vi "database_connection_write_dev_MQTT_database_array.vi"(8 "error in (no error)":errorcluster, 9 "data 2":dbl[](array[numeric]), 10 "Machine Data":T5={"Zload"="", "Yload"="", "Xload"="", "path_position"="", "Fovr"="", "SspeedOvr"="", "Program Name"="", "Program status"="", "Block of code being executed"="", "Line of code"="", "Machine availability"="", "Emergency status"="", "Controller mode"="", "Tool_id"="UNAVAILABLE"}, 11 "current time 2":timestamp) -> (3 "error out":errorcluster)   [LabVIEW 2017]
uses:
  mqtt Folder/src/class/mqtt/mqttTypedef/mqttConnectionStatus.ctl
  mqtt Folder/src/class/mqtt/mqttTypedef/mqttConnectionMeta.ctl
  mqtt Folder/src/class/mqtt/mqttTypedef/mqttQOSlevel.ctl
  data_base_structure.ctl
  mqtt Folder/src/class/mqtt/mqttConfigFunction.ctl
  mqtt Folder/src/class/mqtt/mqttTypedef/mqttBroker.ctl
  mqtt Folder/src/class/mqtt/mqttTypedef/mqttConnectionFlags.ctl
  mqtt Folder/src/class/mqtt/mqttTypedef/mqttWillInformation.ctl
  mqtt Folder/src/class/mqtt/mqttTXqueue/mqttTXdataQueueFunction.ctl
  mqtt Folder/src/class/mqtt/mqttTXqueue/mqttRXsubscriptionEventFunction.ctl
  <vilib>/addons/database/Connection.llb/DB Tools Open Connec (Path).vi
  mqtt Folder/src/class/mqtt/mqtt.lvclass
  <vilib>/addons/database/NI_Database_API.lvlib
panel:
  out "output array 2":dbl[](array[numeric])
  out "output cluster 2":T1
  out "output cluster":cluster{"current time 2":timestamp, dbl}
  out "output array":string[](array[string])
  out "size(s) 2":i32
  out "error out 3":errorcluster
  out "publishSuccess 2":bool=TRUE
  out "publishMessageID 2":u16 format="%02x"
  out "valueSent 2":string="14:19:17.238_"
  in  "connMeta 2":T2
  in  "topic 2":string="a/b"
  out "connStatus 2":T4
  out "sessionPresent 2":bool
  out "data 3":dbl[](array[numeric])
  out "size(s)":i32
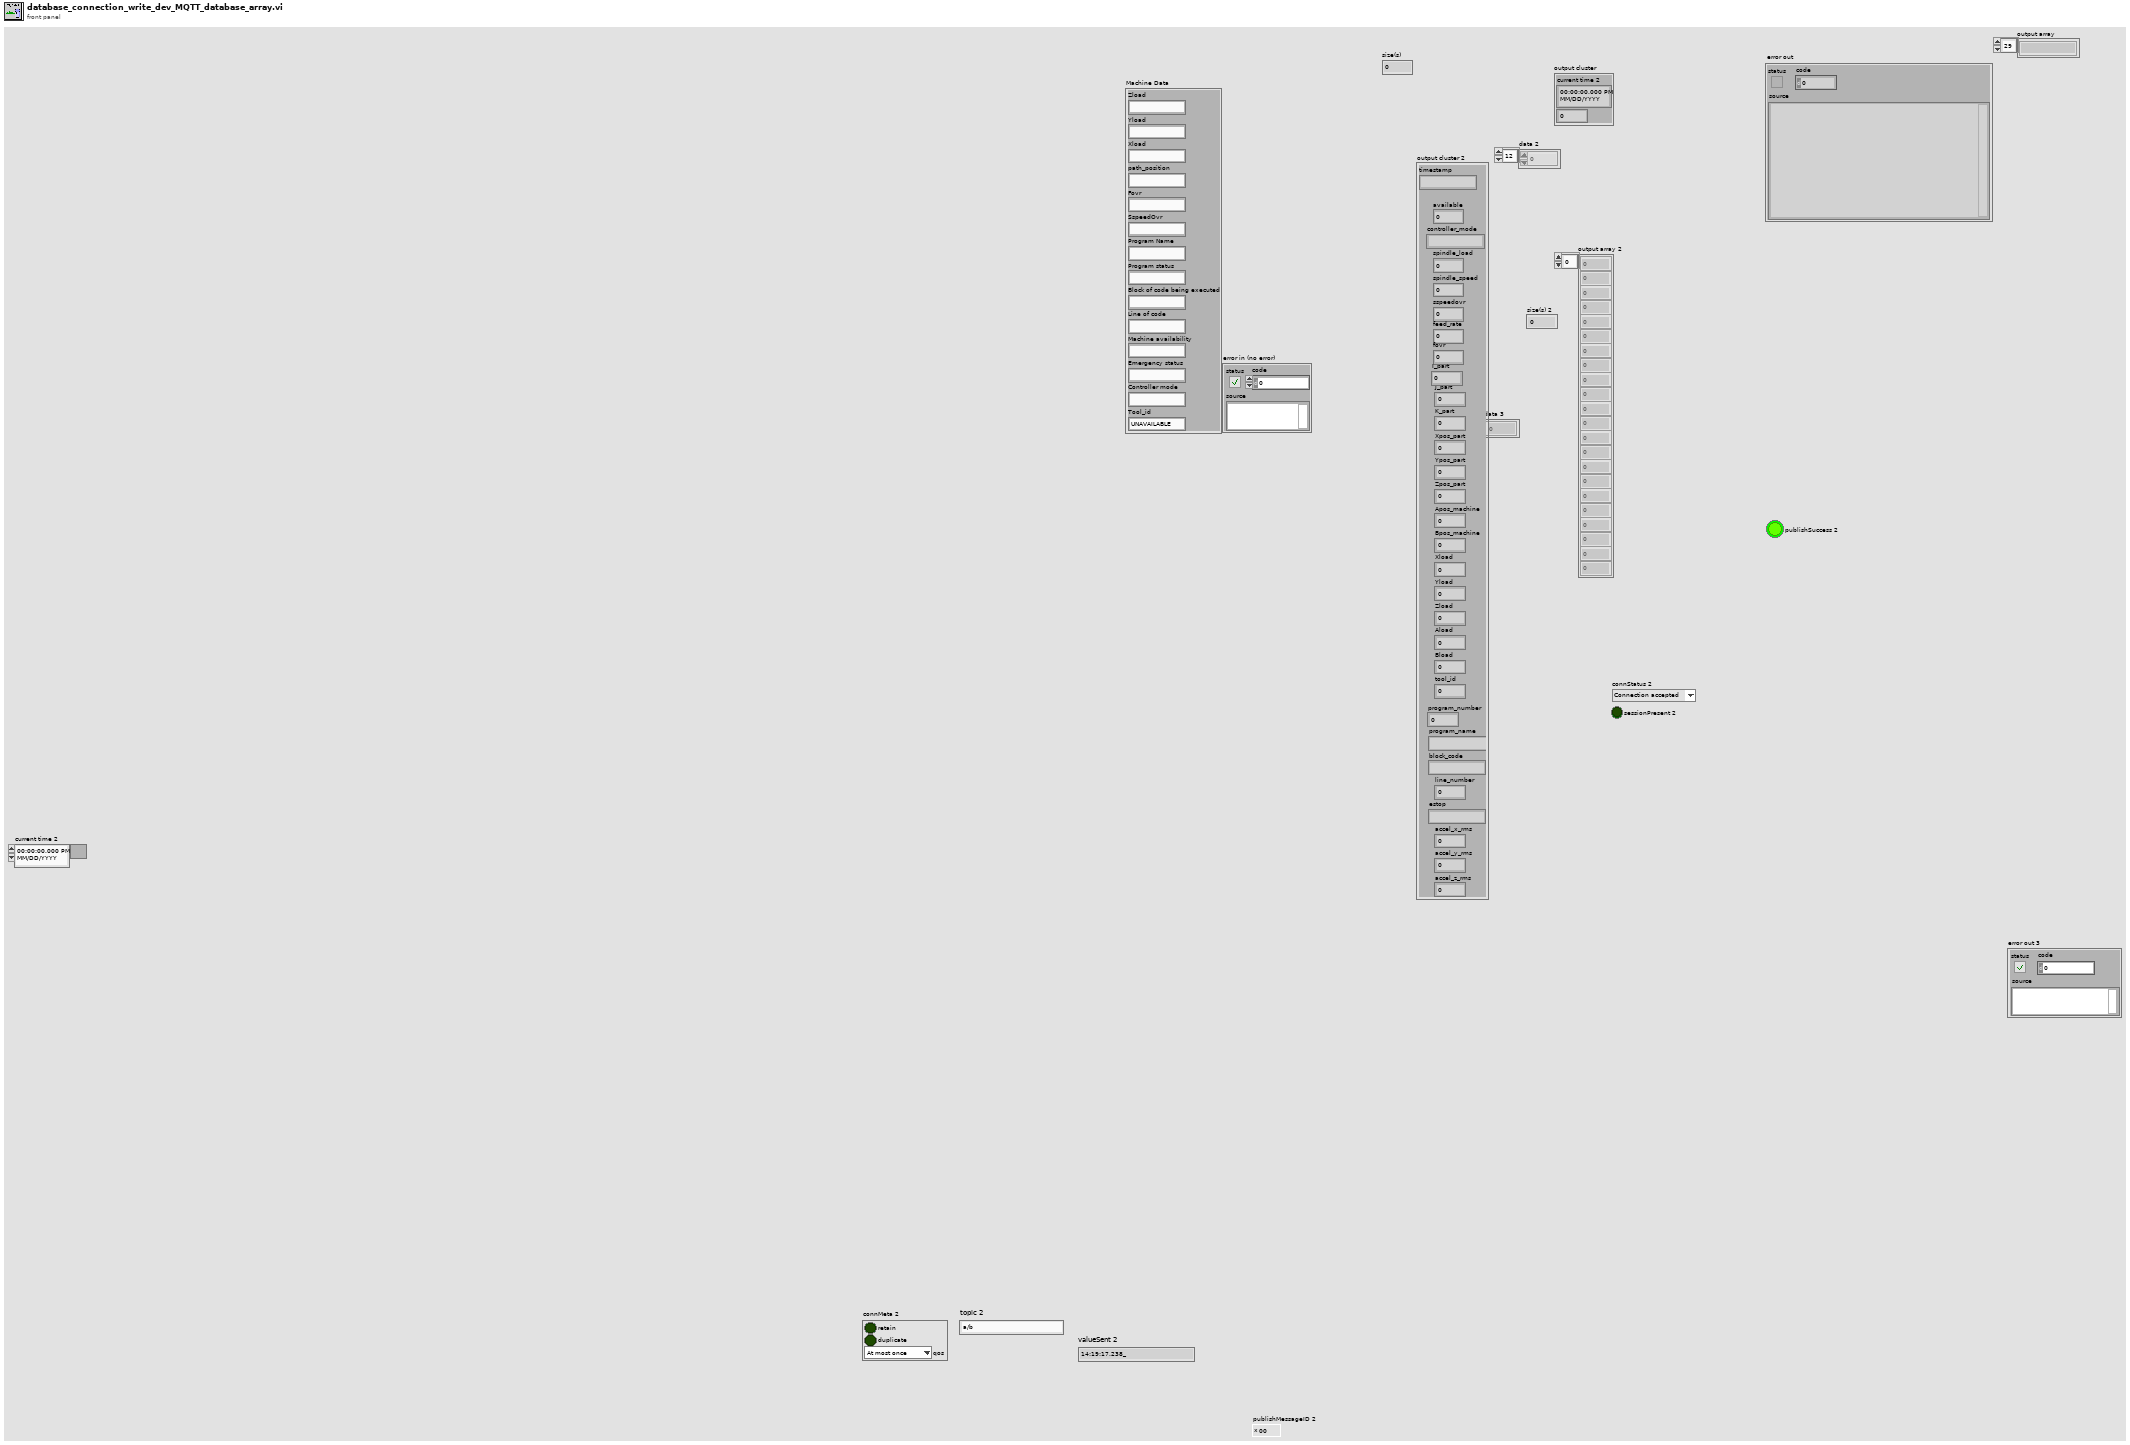
[diagram p1: front panel]
types:
  T1 = typedef "data_base_structure.ctl" = cluster{"available ":dbl, "controller_mode":string, "spindle_load":dbl, "spindle_speed ":dbl, "sspeedovr":dbl, "J_part":dbl, "K_part":dbl, "Xpos_part":dbl, "Ypos_part":dbl, "Zpos_part":dbl, "Apos_machine":dbl, "Bpos_machine":dbl, "Xload":dbl, "Yload":dbl, "Zload":dbl, "Aload":dbl, "Bload":dbl, "tool_id":dbl, "program_name":string, "block_code":string, "line_number":dbl, "estop":string, "accel_x_rms":dbl, "accel_y_rms":dbl, "accel_z_rms":dbl, "program_number":dbl, "timestamp":string, "feed_rate ":dbl, "fovr":dbl, "I_part ":dbl}
  T2 = typedef "mqttConnectionMeta.ctl" = cluster{"retain":bool, "duplicate":bool, "qos":T3}
  T3 = typedef "mqttQOSlevel.ctl" = enum8{"At most once", "At least once", "Exactly once", "Reserved"}
  T4 = typedef "mqttConnectionStatus.ctl" = enum16{"Connection accepted", "Connection refused: unacceptable protocol version", "Connection refused: identifier rejected", "Connection refused: Server unavailable", "Connection refused: bad user name or password", "Connection refused: not authorized"}
  T5 = cluster{"Zload":string, "Yload":string, "Xload":string, "path_position":string, "Fovr":string, "SspeedOvr":string, "Program Name":string, "Program status":string, "Block of code being executed":string, "Line of code":string, "Machine availability":string, "Emergency status":string, "Controller mode":string, "Tool_id":string}
  T6 = typedef "mqttRXsubscriptionEventFunction.ctl" = enum16{"init", "deinit", "getEventRef", "event"}
  T7 = typedef "mqttTXdataQueueFunction.ctl" = enum16{"init", "deinit", "getQueue", "enqueue"}
  T8 = typedef "mqttWillInformation.ctl" = cluster{"User Name":string, "Password":string}
  T9 = typedef "mqttConnectionFlags.ctl" = cluster{"reserved":bool, "clean session":bool, "will flag":bool, "willQOS":enum8{"At most once", "At least once", "Exactly once", "Reserved"}, "will retain":bool, "password":bool, "user name":bool}
  T10 = typedef "mqttBroker.ctl" = cluster{"address":string, "port":u16, "connTimeout":i32, "writeTimeout":i32, "readTimeout":i32, "subTimeout":i32}
  T11 = typedef "mqtt.lvclass/mqttConfigFunction.ctl" = enum16{"init", "deinit", "set", "get"}
  T12 = enum8{"Enabled", "Disabled", "Disabled and Grayed Out"}
  T13 = cluster{"data 2[0]":dbl, "data 2[1]":dbl, "data 2[2]":dbl, "data 2[3]":dbl, "data 2[4]":dbl, "data 2[5]":dbl, "data 2[6]":dbl, "data 2[7]":dbl, "data 2[8]":dbl, "data 2[9]":dbl, "data 2[10]":dbl, "data 2[11]":dbl, "data 2[12]":dbl, "data 2[13]":dbl, "data 2[14]":dbl, "data 2[15]":dbl, "data 2[16]":dbl, "data 2[17]":dbl}
  T14 = cluster{"data 2[0]":dbl, "data 2[1]":dbl, "data 2[2]":dbl, "data 2[3]":dbl, "data 2[4]":dbl, "data 2[5]":dbl, "data 2[6]":dbl, "data 2[7]":dbl, "data 2[8]":dbl, "data 2[9]":dbl, "data 2[10]":dbl, "data 2[11]":dbl, "data 2[12]":dbl, "data 2[13]":dbl, "data 2[14]":dbl, "data 2[15]":dbl, "data 2[16]":dbl, "data 2[17]":dbl, "data 2[18]":dbl, "data 2[19]":dbl, "data 2[20]":dbl, "data 2[21]":dbl}
  T15 = typedef "NI_Database_API.lvlib/Conn ObjectReference.ctl" = refnum<k1>
  T16 = cluster{"date/time string":string, dbl, "Controller mode":string, "data 2[0]":dbl, "data 2[1]":dbl, "data 2[2]":dbl, "data 2[3]":dbl, "data 2[4]":dbl, "data 2[5]":dbl, "data 2[6]":dbl, "data 2[7]":dbl, "data 2[8]":dbl, "data 2[9]":dbl, "data 2[10]":dbl, "data 2[11]":dbl, "data 2[12]":dbl, "data 2[13]":dbl, "data 2[14]":dbl, "data 2[15]":dbl, "data 2[16]":dbl, "data 2[17]":dbl, dbl, "data 2[18]":dbl, "Program Name":string, "Block of code being executed":string, dbl, "Emergency status":string, "data 2[20]":dbl, "data 2[19]":dbl, "data 2[21]":dbl}
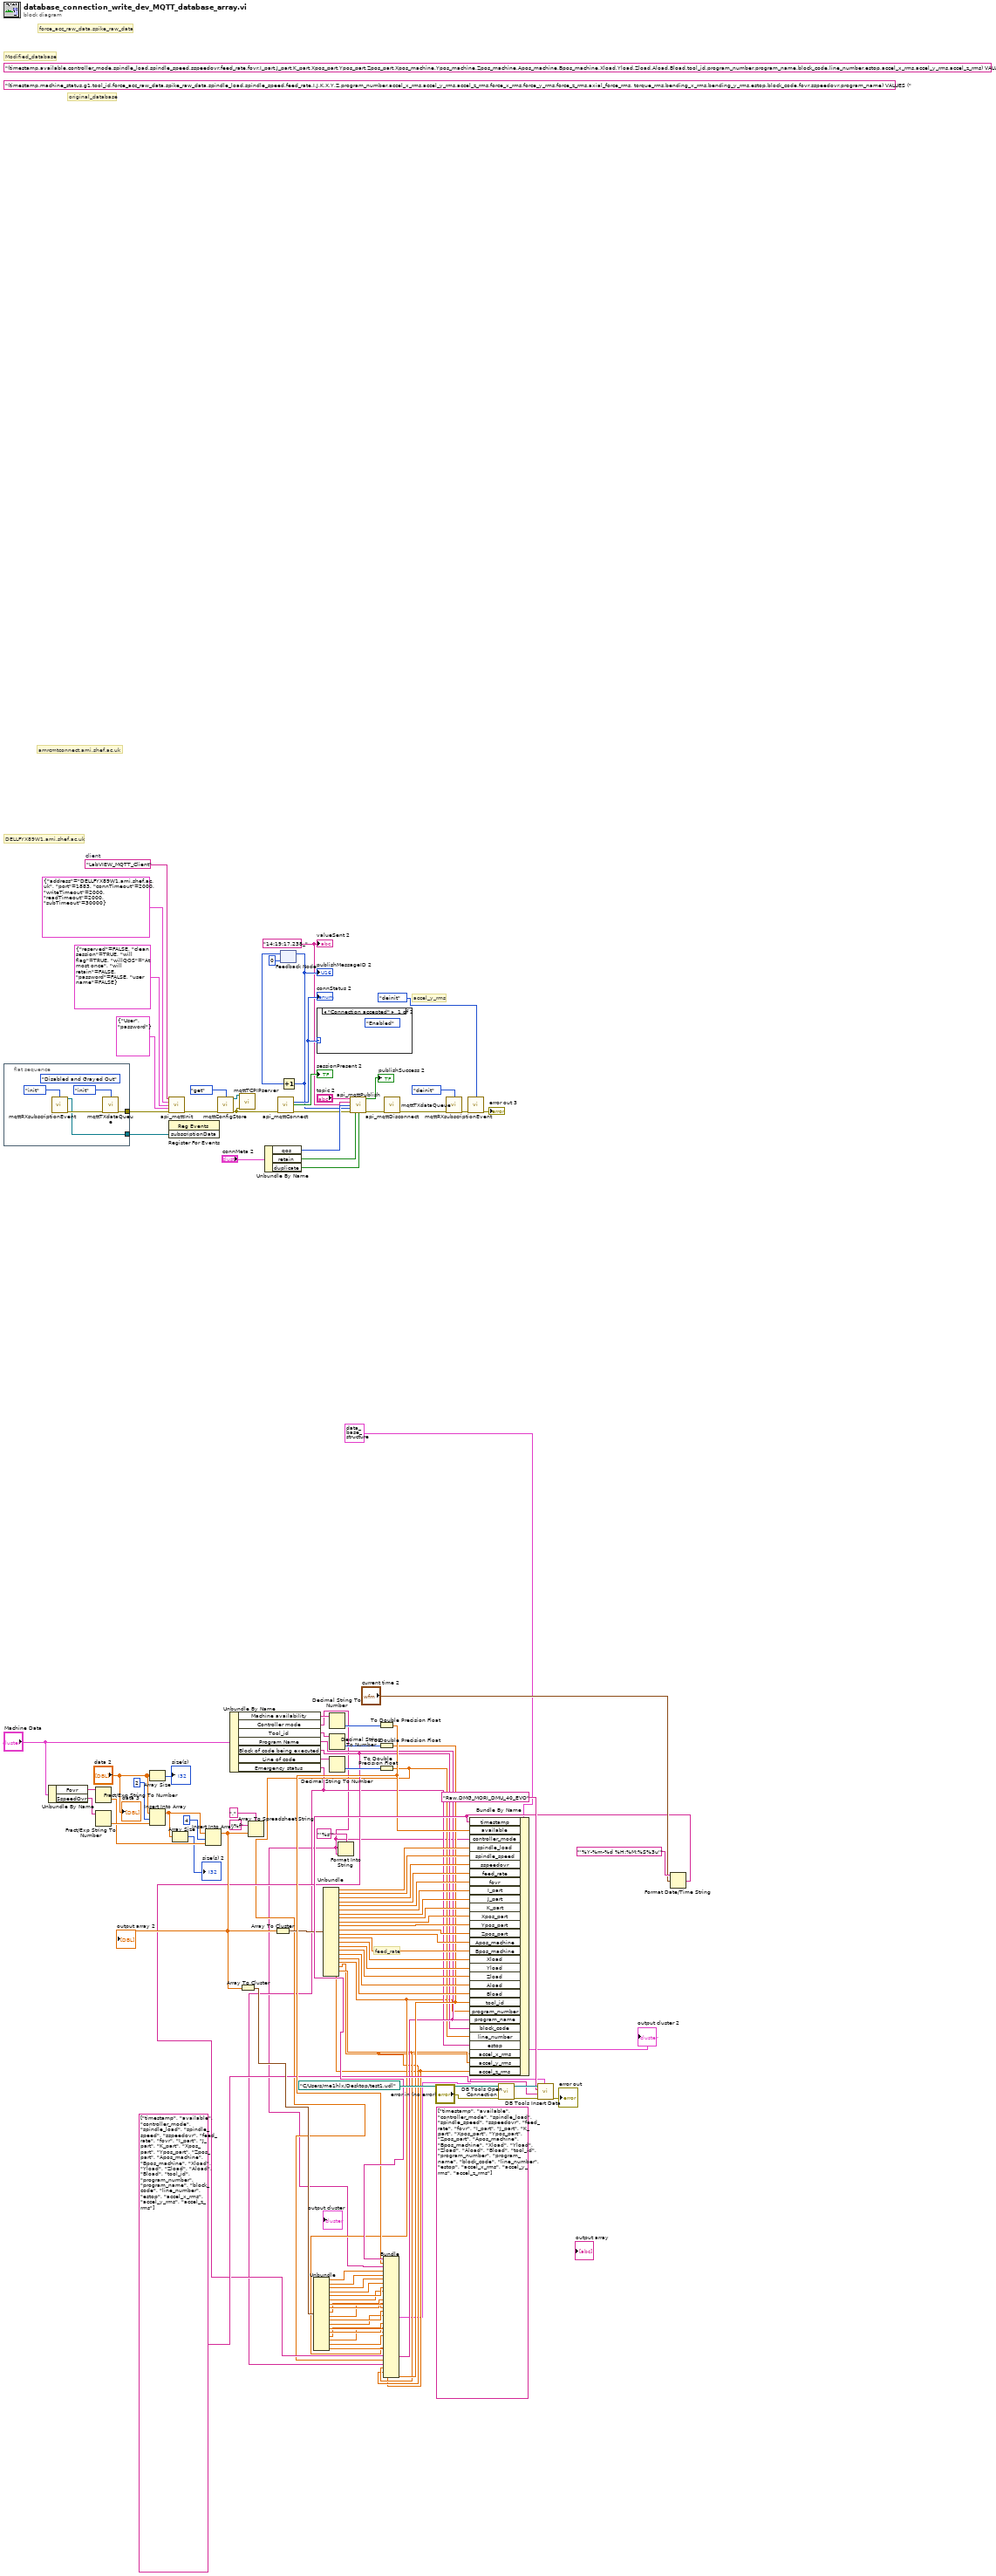
[diagram p0: block diagram]
diagram:
  (unwired) string[] ["timestamp", "available", "controller_mode", "spindle_load", "spindle_speed", "sspeedovr", "feed_rate", "fovr", "I_part", "J_part", "K_part", "Xpos_part", "Ypos_part", "Zpos_part", "Apos_machine", "Bpos_machine", "Xload", "Yload", "Zload", "Aload", "Bload", "tool_id", "program_number", "program_name", "block_code", "line_number", "estop", "accel_x_rms", "accel_y_rms", "accel_z_rms"]
  w71 = "14:19:17.238_" ("valueSent 2")
  (unwired) "(timestamp,available,controller_mode,spindle_load,spindle_speed,sspeedovr,feed_rate,fovr,I_part,J_part,K_part,Xpos_part,Ypos_part,Zpos_part,Xpos_machine,Ypos_machine,Zpos_machine,Apos_machine,Bpos_machine,Xload,Yload,Zload,Aload,Bload,tool_id,program_number,program_name,block_code,line_number,estop,accel_x_rms,accel_y_rms,accel_z_rms) VALUES (" ("string")
  w104 = "LabVIEW_MQTT_Client"  # client
  (unwired) "(timestamp,machine_status,g1,tool_id,force_acc_raw_data,spike_raw_data,spindle_load,spindle_speed,feed_rate,I,J,K,X,Y,Z,program_number,accel_x_rms,accel_y_rms,accel_z_rms,force_x_rms,force_y_rms,force_z_rms,axial_force_rms, torque_rms,bending_x_rms,bending_y_rms,estop,block_code,fovr,sspeedovr,program_name) VALUES (" ("string")
  # "accel_y_rms"
  # "feed_rate"
  # "original_database"
  # "force_acc_raw_data,spike_raw_data"
  # "Modified_database"
  # "amrcmtconnect.ami.shef.ac.uk"
  # "DELLFYX89W1.ami.shef.ac.uk"
  n1 = flat-sequence {
    tunnel: [w116] -> w109
    tunnel: [w113] -> w105
    frame #0 {
      (unwired) T12."Disabled and Grayed Out" ("Disabled")
      n2 = call "mqttRXsubscriptionEvent.vi"("function"=mqttRXsubscriptionEventFunction."init") -> ("subscriptionData"=w113:refnum<user-event>, "error out"=w115:errorcluster)  [unwired: 13 in]
      n3 = call "mqttTXdataQueue.vi"("function"=mqttTXdataQueueFunction."init", "error in (no error)"=w115) -> ("error out"=w116:errorcluster)  [unwired: 12 in, 1 out]
    }
  }
  n4 = Unbundle By Name("Machine Data") -> ("Fovr"=w75:string, "SspeedOvr"=w80:string)
  n5 = Fract/Exp String To Number(string=w75) -> (number=w77:dbl)  [unwired: 3 in, 1 out]
  n6 = Fract/Exp String To Number(string=w80) -> (number=w79:dbl)  [unwired: 3 in, 1 out]
  n7 = Array Size(array="data 2") -> (size(s)=→"size(s)":i32)
  n8 = Insert Into Array(array="data 2", index=2, new element=w79) -> (w67:dbl[])
  n9 = call "api_mqttInit.vi"("client"=w104, "broker"=T10 {"address"="DELLFYX89W1.ami.shef.ac.uk", "port"=1883, "connTimeout"=2000, "writeTimeout"=2000, "readTimeout"=2000, "subTimeout"=30000}, "connFlags"=T9 {"reserved"=FALSE, "clean session"=TRUE, "will flag"=TRUE, "willQOS"=enum."At most once", "will retain"=FALSE, "password"=FALSE, "user name"=FALSE}, "User Info"=T8 {"User Name"="User", "Password"="password"}, "error in (no error)"=w109) -> ("error out"=w107:errorcluster)  [unwired: 10 in]
  n10 = register-events(w105) -> ()  [unwired: 2 in, 2 out]
  n11 = Array Size(array=w67) -> (size(s)=→"size(s) 2":i32)
  n12 = Insert Into Array(array=w67, index=4, new element=w77) -> (w30:dbl[])
  "output array 2" <- w30
  n13 = call "mqttConfigStore.vi"("function"=mqttConfigFunction."get", "error in (no error)"=w107) -> ("mqtt.lvclass out"=w106:refnum<class "mqtt.lvclass">, "error out"=w98:errorcluster)  [unwired: 12 in]
  n14 = Unbundle By Name("Machine Data") -> ("Machine availability"=w40:string, "Controller mode"=w3:string, "Tool_id"=w62:string, "Program Name"=w11:string, "Block of code being executed"=w10:string, "Line of code"=w61:string, "Emergency status"=w8:string)
  n15 = call "mqttTCPIPserver.vi"("mqtt.lvclass"=w106, "error in (no error)"=w98) -> ()  [unwired: 12 in, 2 out]
  n16 = Array To Cluster(array=w30) -> (cluster=w29:T13)
  n17 = Array To Spreadsheet String(delimiter (Tab)=",", array=w30, 3:"%f" ("format string")) -> ()  [unwired: 1 out]
  n18 = Unbundle By Name("connMeta 2") -> ("qos"=w95:T3, "retain"=w94:bool, "duplicate"=w93:bool)
  n19 = Array To Cluster(array=w30) -> (cluster=w34:T14)
  n20 = call "api_mqttConnect.vi"("error in (no error)"=w98) -> ("connStatus"=w100:T4, "sessionPresent"=→"sessionPresent 2":bool, "error out"=w92:errorcluster)  [unwired: 11 in, 1 out]
  "connStatus 2" <- w100
  n21 = feedback #1(u16 0) -> (w90:u16)
  n22 = Increment(x=w90) -> (x+1=w89:u16)
  "publishMessageID 2" <- w89
  n23 = feedback-in #1(w89) -> ()
  n24 = Unbundle(w29) -> ("data 2[0]"=w33:dbl, "data 2[1]"=w32:dbl, "data 2[2]"=w31:dbl, "data 2[3]"=w28:dbl, "data 2[4]"=w26:dbl, "data 2[5]"=w25:dbl, "data 2[6]"=w24:dbl, "data 2[7]"=w23:dbl, "data 2[8]"=w22:dbl, "data 2[9]"=w21:dbl, "data 2[10]"=w20:dbl, "data 2[11]"=w19:dbl, "data 2[12]"=w18:dbl, "data 2[13]"=w17:dbl, "data 2[14]"=w16:dbl, "data 2[15]"=w15:dbl, "data 2[16]"=w14:dbl, "data 2[17]"=w13:dbl)
  n25 = case shown="\"Connection accepted\"" w100 {
    frame "Connection accepted" {
      (unwired) T12."Enabled" ("Disabled")
    }
    frame Default {
    }
  }
  n26 = Unbundle(w34) -> ("data 2[0]"=w57:dbl, "data 2[1]"=w56:dbl, "data 2[2]"=w55:dbl, "data 2[3]"=w54:dbl, "data 2[4]"=w53:dbl, "data 2[5]"=w52:dbl, "data 2[6]"=w51:dbl, "data 2[7]"=w50:dbl, "data 2[8]"=w49:dbl, "data 2[9]"=w48:dbl, "data 2[10]"=w47:dbl, "data 2[11]"=w46:dbl, "data 2[12]"=w45:dbl, "data 2[13]"=w44:dbl, "data 2[14]"=w66:dbl, "data 2[15]"=w43:dbl, "data 2[16]"=w65:dbl, "data 2[17]"=w42:dbl, "data 2[18]"=w7:dbl, "data 2[19]"=w5:dbl, "data 2[20]"=w6:dbl, "data 2[21]"=w4:dbl)
  n27 = Decimal String To Number(string=w40) -> (number=w39:i32)  [unwired: 2 in, 1 out]
  n28 = Decimal String To Number(string=w62) -> (number=w63:i32)  [unwired: 2 in, 1 out]
  n29 = Decimal String To Number(string=w61) -> (number=w60:i32)  [unwired: 2 in, 1 out]
  n30 = Format Into String(format string="'%s'", w3) -> ()  [unwired: 2 in, 2 out]
  n31 = call "api_mqttPublish.vi"("topic"="topic 2", "value"=w71, "QoS (At most once)"=w95, "messageID"=w89, "error in (no error)"=w92, "retain(F)"=w94, "duplicate(F)"=w93) -> ("success"=→"publishSuccess 2":bool, "error out"=w82:errorcluster)  [unwired: 7 in]
  n32 = To Double Precision Float(number=w39) -> (double precision float=w36:dbl)
  n33 = To Double Precision Float(number=w63) -> (double precision float=w12:dbl)
  n34 = To Double Precision Float(number=w60) -> (double precision float=w9:dbl)
  n35 = call "api_mqttDisconnect.vi"("error in (no error)"=w82) -> ("error out"=w86:errorcluster)  [unwired: 13 in, 1 out]
  n36 = call "mqttTXdataQueue.vi"("function"=mqttTXdataQueueFunction."deinit", "error in (no error)"=w86) -> ("error out"=w84:errorcluster)  [unwired: 12 in, 1 out]
  n37 = call "mqttRXsubscriptionEvent.vi"("function"=mqttRXsubscriptionEventFunction."deinit", "error in (no error)"=w84) -> ("error out"=→"error out 3":errorcluster)  [unwired: 12 in, 1 out]
  n38 = call-poly <vilib>:"DB Tools Open Connection.vi"("error in (no error)"="error in (no error)", "connection information"=path "C:/Users/me1hlx/Desktop/test1.udl") -> ("error out"=w64:errorcluster, "connection reference"=w72:T15)  [unwired: 6 in]
  n39 = Format Date/Time String(time format string (%c)="'%Y-%m-%d %H:%M:%S%3u'", seconds (now)="current time 2") -> (date/time string=w37:string)  [unwired: 1 in]
  n40 = Bundle("date/time string"=w37, w36, "Controller mode"=w3, "data 2[0]"=w33, "data 2[1]"=w32, "data 2[2]"=w31, "data 2[3]"=w28, "data 2[4]"=w26, "data 2[5]"=w25, "data 2[6]"=w24, "data 2[7]"=w23, "data 2[8]"=w22, "data 2[9]"=w21, "data 2[10]"=w20, "data 2[11]"=w19, "data 2[12]"=w18, "data 2[13]"=w17, "data 2[14]"=w16, "data 2[15]"=w15, "data 2[16]"=w14, "data 2[17]"=w13, w12, "data 2[18]"=w7, "Program Name"=w11, "Block of code being executed"=w10, w9, "Emergency status"=w8, "data 2[20]"=w6, "data 2[19]"=w5, "data 2[21]"=w4) -> (w1:T16)  [unwired: 1 in]
  n41 = Bundle By Name(cluster=T1 {"available "=0.0, "controller_mode"="", "spindle_load"=0.0, "spindle_speed "=0.0, "sspeedovr"=0.0, "J_part"=0.0, "K_part"=0.0, "Xpos_part"=0.0, "Ypos_part"=0.0, "Zpos_part"=0.0, "Apos_machine"=0.0, "Bpos_machine"=0.0, "Xload"=0.0, "Yload"=0.0, "Zload"=0.0, "Aload"=0.0, "Bload"=0.0, "tool_id"=0.0, "program_name"="", "block_code"="", "line_number"=0.0, "estop"="", "accel_x_rms"=0.0, "accel_y_rms"=0.0, "accel_z_rms"=0.0, "program_number"=0.0, "timestamp"="", "feed_rate "=0.0, "fovr"=0.0, "I_part "=0.0} ("Cluster"), "timestamp"=w37, "available"=w36, "controller_mode"=w3, "spindle_load"=w57, "spindle_speed"=w56, "sspeedovr"=w55, "feed_rate"=w54, "fovr"=w53, "I_part"=w52, "J_part"=w51, "K_part"=w50, "Xpos_part"=w49, "Ypos_part"=w48, "Zpos_part"=w47, "Apos_machine"=w46, "Bpos_machine"=w45, "Xload"=w44, "Yload"=w66, "Zload"=w43, "Aload"=w65, "Bload"=w42, "tool_id"=w12, "program_number"=w7, "program_name"=w11, "block_code"=w10, "line_number"=w9, "estop"=w8, "accel_x_rms"=w5, "accel_y_rms"=w6, "accel_z_rms"=w4) -> (→"output cluster 2":T1)
  n42 = call <vilib>:"DB Tools Insert Data.vi"("data"=w1, "error in (no error)"=w64, "columns"=string[] ["timestamp", "available", "controller_mode", "spindle_load", "spindle_speed", "sspeedovr", "feed_rate", "fovr", "I_part", "J_part", "K_part", "Xpos_part", "Ypos_part", "Zpos_part", "Apos_machine", "Bpos_machine", "Xload", "Yload", "Zload", "Aload", "Bload", "tool_id", "program_number", "program_name", "block_code", "line_number", "estop", "accel_x_rms", "accel_y_rms", "accel_z_rms"], "table"="Raw.DMG_MORI_DMU_40_EVO" ("string"), "connection reference"=w72) -> ("error out"=→"error out":errorcluster)  [unwired: 5 in, 1 out]
  "data 3" <- "data 2"
  "valueSent 2" <- w71
